vi "Embed VI Subpanel.vi"(8 "Error In":errorcluster, 10 "VI Ref":refnum<vi>, 11 "Subpanel Ref":refnum<vi>) -> (0 "Error Out":errorcluster)   [LabVIEW 2015]
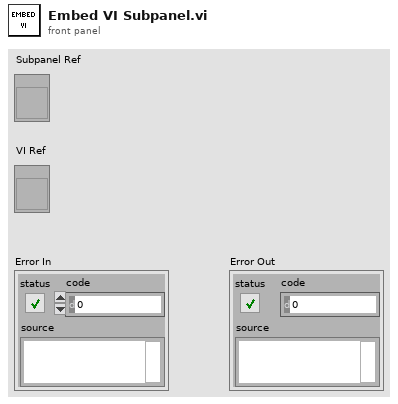
[diagram p1: front panel]
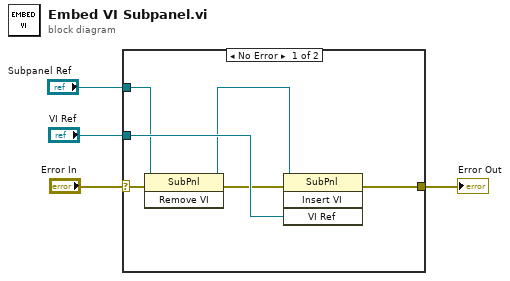
[diagram p0: block diagram]
diagram:
  n1 = case shown="No Error" "Error In" {
    selector: "Error In" -> [w8 w11]
    tunnel: [w9 w11] -> w3
    tunnel: "VI Ref" -> [w10 _]
    tunnel: "Subpanel Ref" -> [w7 _]
    frame No Error {
      n2 = invoke class="SubPnl" method="Remove VI"(reference=w7, error in=w8) -> (reference out=w6:refnum<vi>, error out=w5:errorcluster)  [unwired: 1 in, 1 out]
      n3 = invoke class="SubPnl" method="Insert VI"(reference=w6, error in=w5, "VI Ref"=w10) -> (error out=w9:errorcluster)  [unwired: 1 in, 3 out]
    }
    frame Error {
    }
  }
  "Error Out" <- w3
